vi "tcp multi read async setup.vi"(8 "error in (no error)":errorcluster, 11 "TCP Ports":refnum<k5>[](array[refnum])) -> (0 "error out":errorcluster, 2 "time for vi":u32, 3 "VIout":refnum<vi>)   [LabVIEW 2013]
panel:
  out "NaN/Path/Refnum? 3":bool
  out "NaN/Path/Refnum? 2":bool
  out "NaN/Path/Refnum?":bool
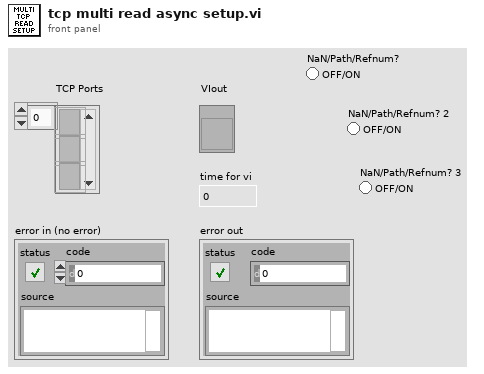
[diagram p1: front panel]
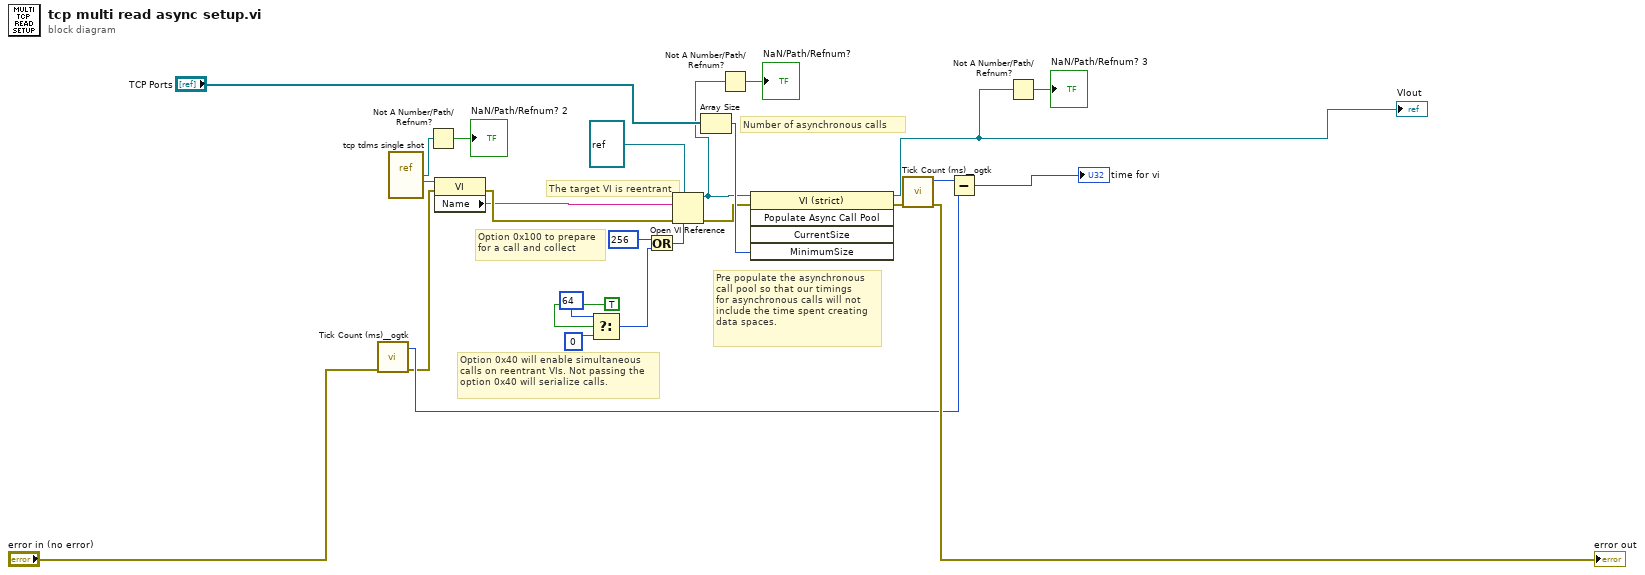
[diagram p0: block diagram]
diagram:
  # "Pre populate the asynchronous\ncall pool so that our timings\nfor asynchronous calls will not\ninclude the time spent creating\ndata spaces."
  # "The target VI is reentrant"
  # "Number of asynchronous calls"
  # "Option 0x40 will enable simultaneous\ncalls on reentrant VIs. Not passing the\noption 0x40 will serialize calls."
  # "Option 0x100 to prepare\nfor a call and collect"
  n1 = call <userlib>:"Tick Count (ms)__ogtk.vi"("error in (no error)"="error in (no error)") -> ("error out"=w18:errorcluster, "millisecond timer value"=w22:u32)  [unwired: 9 in]
  n2 = vi-ref "tcp tdms single shot.vi"() -> (w3:refnum<vi>)
  n3 = Not A Number/Path/Refnum?(number/path/refnum=w3) -> (NaN/Path/Refnum?=→"NaN/Path/Refnum? 2":bool)
  n4 = property class="VI"(reference=w3, error in=w18) -> (error out=w25:errorcluster, "Name"=w8:string)  [unwired: 1 out]
  n5 = Select(t=64 ("options"), s=TRUE ("x40 to parallelize!!"), f=0 ("options")) -> (s? t:f=w14:i32)
  n6 = Or(x=256 ("options"), y=w14) -> (x .or. y?=w11:i32)
  n7 = Open VI Reference(type specifier VI Refnum (for type only)=refnum<vi> refnum, vi path=w8, options=w11, error in (no error)=w25) -> (vi reference=w6:refnum<vi>, error out=w15:errorcluster)  [unwired: 2 in]
  n8 = Array Size(array="TCP Ports") -> (size(s)=w17:i32)
  n9 = Not A Number/Path/Refnum?(number/path/refnum=w6) -> (NaN/Path/Refnum?=→"NaN/Path/Refnum?":bool)
  n10 = invoke class="VI (strict)" method="Populate Async Call Pool"(reference=w6, error in=w15, "MinimumSize"=w17) -> (reference out=w1:refnum<vi>, error out=w19:errorcluster)  [unwired: 2 in, 3 out]
  "VIout" <- w1
  n11 = call <userlib>:"Tick Count (ms)__ogtk.vi"("error in (no error)"=w19) -> ("error out"=→"error out":errorcluster, "millisecond timer value"=w21:u32)  [unwired: 9 in]
  n12 = Subtract(x=w21, y=w22) -> (x-y=→"time for vi":u32)
  n13 = Not A Number/Path/Refnum?(number/path/refnum=w1) -> (NaN/Path/Refnum?=→"NaN/Path/Refnum? 3":bool)
